vi "Analog DAQ_Connect.vi"(0 "Instance Inbox Address":string, 11 "error in (no error)":errorcluster) -> (4 "Analog DAQ Out":refnum<class "Analog DAQ.lvclass">, 15 "error out":errorcluster)   [LabVIEW 2013, in "Analog DAQ.lvclass"]
uses:
  Analog DAQ.lvclass
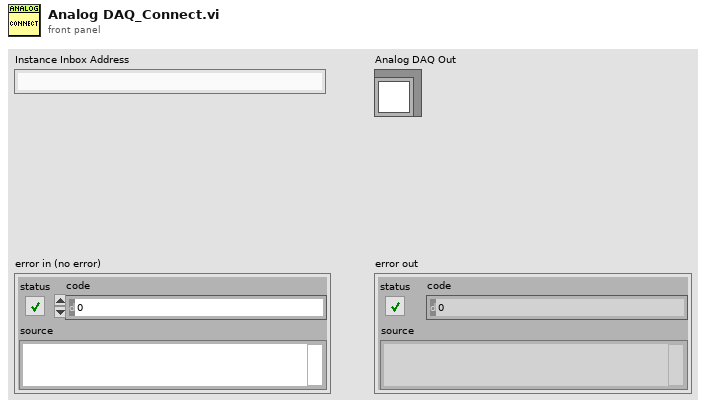
[diagram p1: front panel]
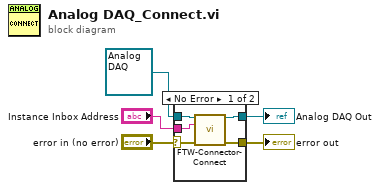
[diagram p0: block diagram]
diagram:
  n1 = case shown="No Error" "error in (no error)" {
    selector: "error in (no error)" -> [w8 w11]
    tunnel: refnum<class "Analog DAQ.lvclass"> refnum ("Actor Template In") -> [w10 w12]
    tunnel: [w9 w12] -> w3
    tunnel: [w7 w11] -> w2
    tunnel: "Instance Inbox Address" -> [w6 _]
    frame No Error {
      n2 = call-dynamic "FTW-Connector-Connect.vi"("FTW Actor Connector Type"=w10, "Instance Inbox Address"=w6, "error in"=w8) -> ("FTW Actor Connector"=w9:refnum<class "Analog DAQ.lvclass">, "error out"=w7:errorcluster)  [unwired: 11 in]
    }
    frame Error {
    }
  }
  "Analog DAQ Out" <- w3
  "error out" <- w2
